vi "Read Force Measured.vi"(11 "ForceSensor in":refnum<class "ForceSensor.lvclass">) -> (2 "Force Demand":T1 format="%.1f", 3 "ForceSensor out":refnum<class "ForceSensor.lvclass">)   [LabVIEW 2013, in "ForceSensor.lvclass"]
uses:
  ForceSensor.lvclass
  Typedefs/ForceDemand.ctl
  ForceSensor.lvclass/ForceSensor.ctl
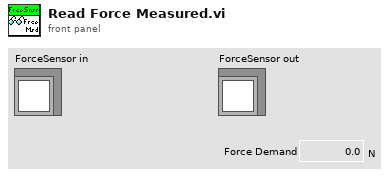
[diagram p1: front panel]
types:
  T1 = typedef "ForceDemand.ctl" = dbl[unit]
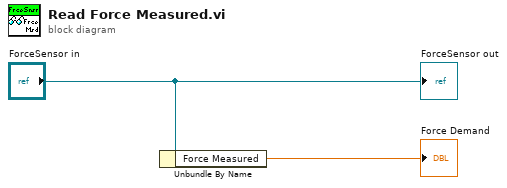
[diagram p0: block diagram]
diagram:
  n1 = Unbundle By Name("ForceSensor in") -> ("Force Measured"=→"Force Demand":T1)
  "ForceSensor out" <- "ForceSensor in"
